vi "x410_test_host_main.vi"() -> ()   [LabVIEW 2025]
uses:
  FPGA/DataMode.ctl
  Host/Output scale.ctl
  <instrlib>/_niInstr/DSP/v1/Shared/Public/IQ Gain.ctl
  <vilib>/FPGAPlugInAG/USRP-X410/niLvFpga_Open_USRP-X410.vi
  <vilib>/rvi/interface/common/dynamic/niFpgaDynamicAddResources.vi
  <vilib>/Utility/error.llb/Error Cluster From Error Code.vi
  <vilib>/rvi/errors/niLvFpgaAdjustHostInterfaceError.vi
  <vilib>/FPGAPlugInAG/Dynamic/niLvFpga_Close_Dynamic.vi
  <vilib>/rvi/interface/nirviOpenFPGA/nirviOpenFPGA.xnode
  FPGA Bitfiles/x410_test_fpga_simple_nJrd0BX6ZCE.lvbitx
  <vilib>/rvi/interface/nirviMethod/nirviMethod.xnode
  <vilib>/rvi/interface/nirviReadWriteControl/nirviReadWriteControl.xnode
  <vilib>/rvi/interface/nirviCloseFPGA/nirviCloseFPGA.xnode
  <vilib>/rvi/errors/niLvFpgaMergeErrorWithErrorCode.vi
  NiFpgaLv.dll
  <vilib>/rvi/interface/Simulation/niFpgaSimulationCallBeginRW.vi
  <vilib>/FPGAPlugInAG/Dynamic/niLvFpga_ReadFifo_Dynamic.vi
  <instrlib>/_niInstr/DSP/v1/Shared/niInstr DSP v1 Shared.lvlib
panel:
  out "Trx Coerced Carrier Frequency":dbl format="%#_8p"
  in  "Trx Carrier Frequency":dbl format="%#_8p"
  in  "Simulated freq (kHz)":dbl
  in  "Host scale":T1
  in  "Mode":T2
  in  "Gain dB":dbl
  out "Waveform Graph":dbl[][](graph)
  out "Done":bool
  out "Init":bool
  in  "# samples to read":u32=16384
  in  "Read":bool
  in  "stop":bool
  out "Coerced Carrier Frequency":dbl=100000.0 format="%#_8p"
  in  "Carrier Frequency":dbl=2000000000.0 format="%#_8p"
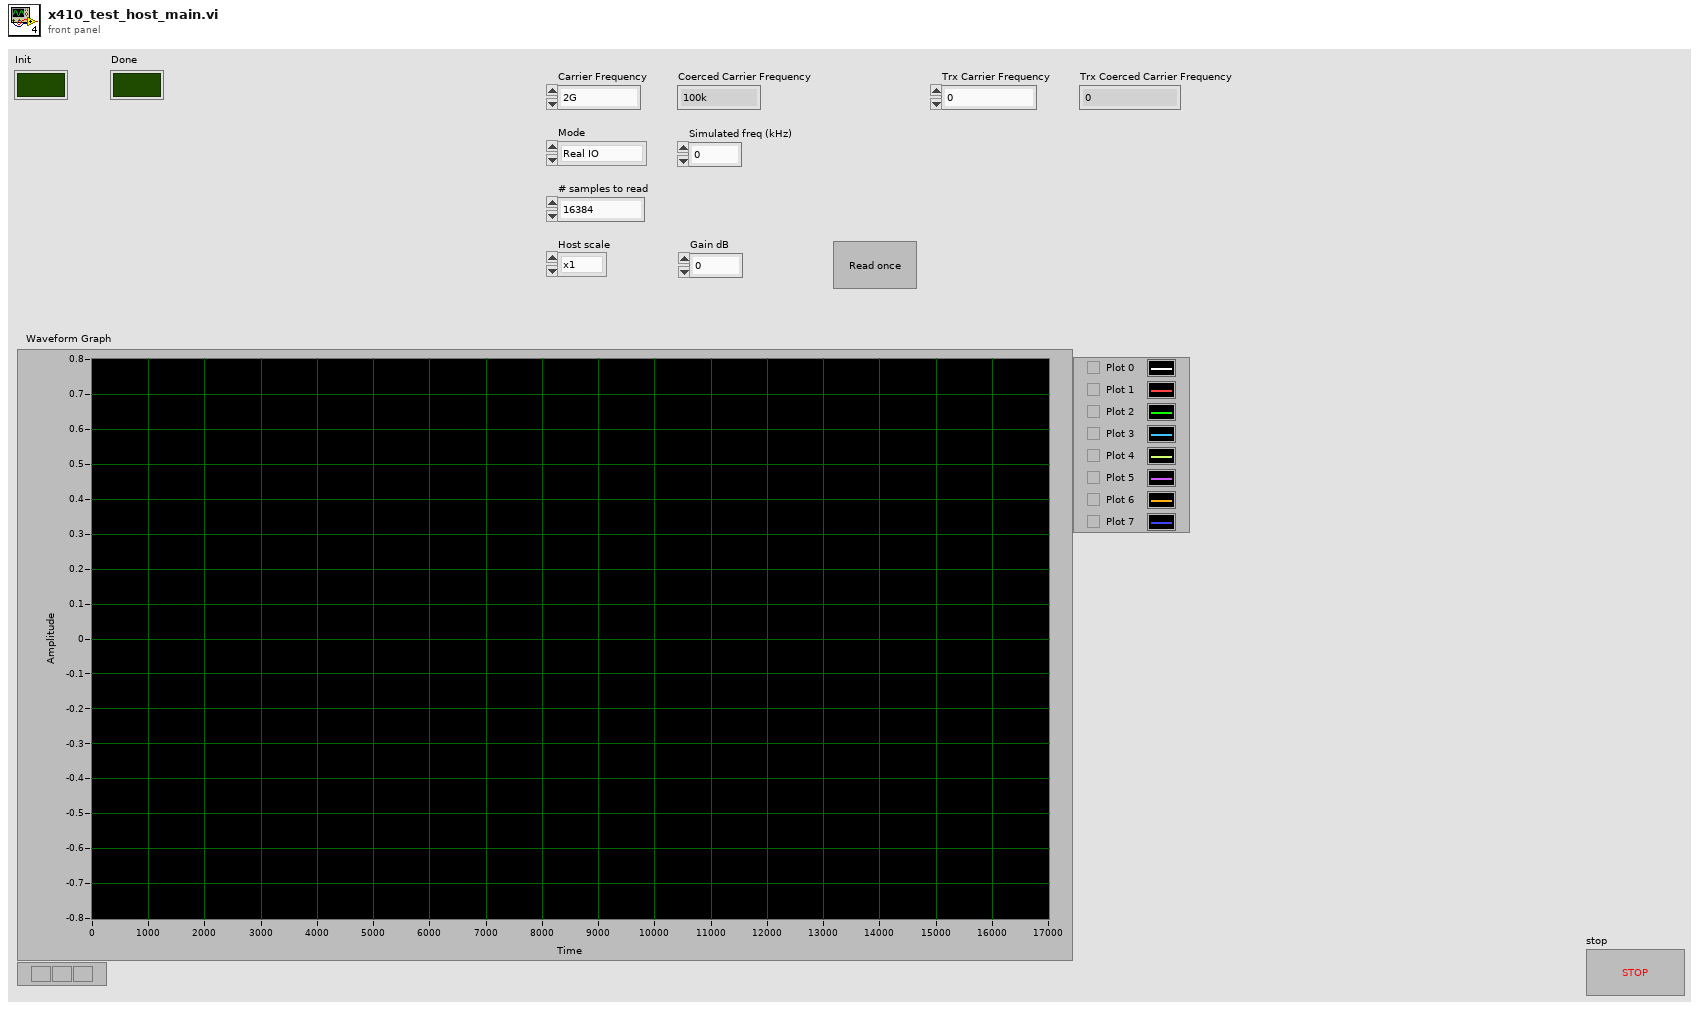
[diagram p1: front panel]
types:
  T1 = typedef "Output scale.ctl" = enum16{"x1", "x2", "x4", "x8", "x16", "x32"}
  T2 = typedef "DataMode.ctl" = enum16{"Real IO", "Simulated"}
  T3 = typedef "niInstr DSP v1 Shared.lvlib/IQ Gain.ctl" = cluster{"gain I":fxp<+/-,24,3>, "gain Q":fxp<+/-,24,3>}
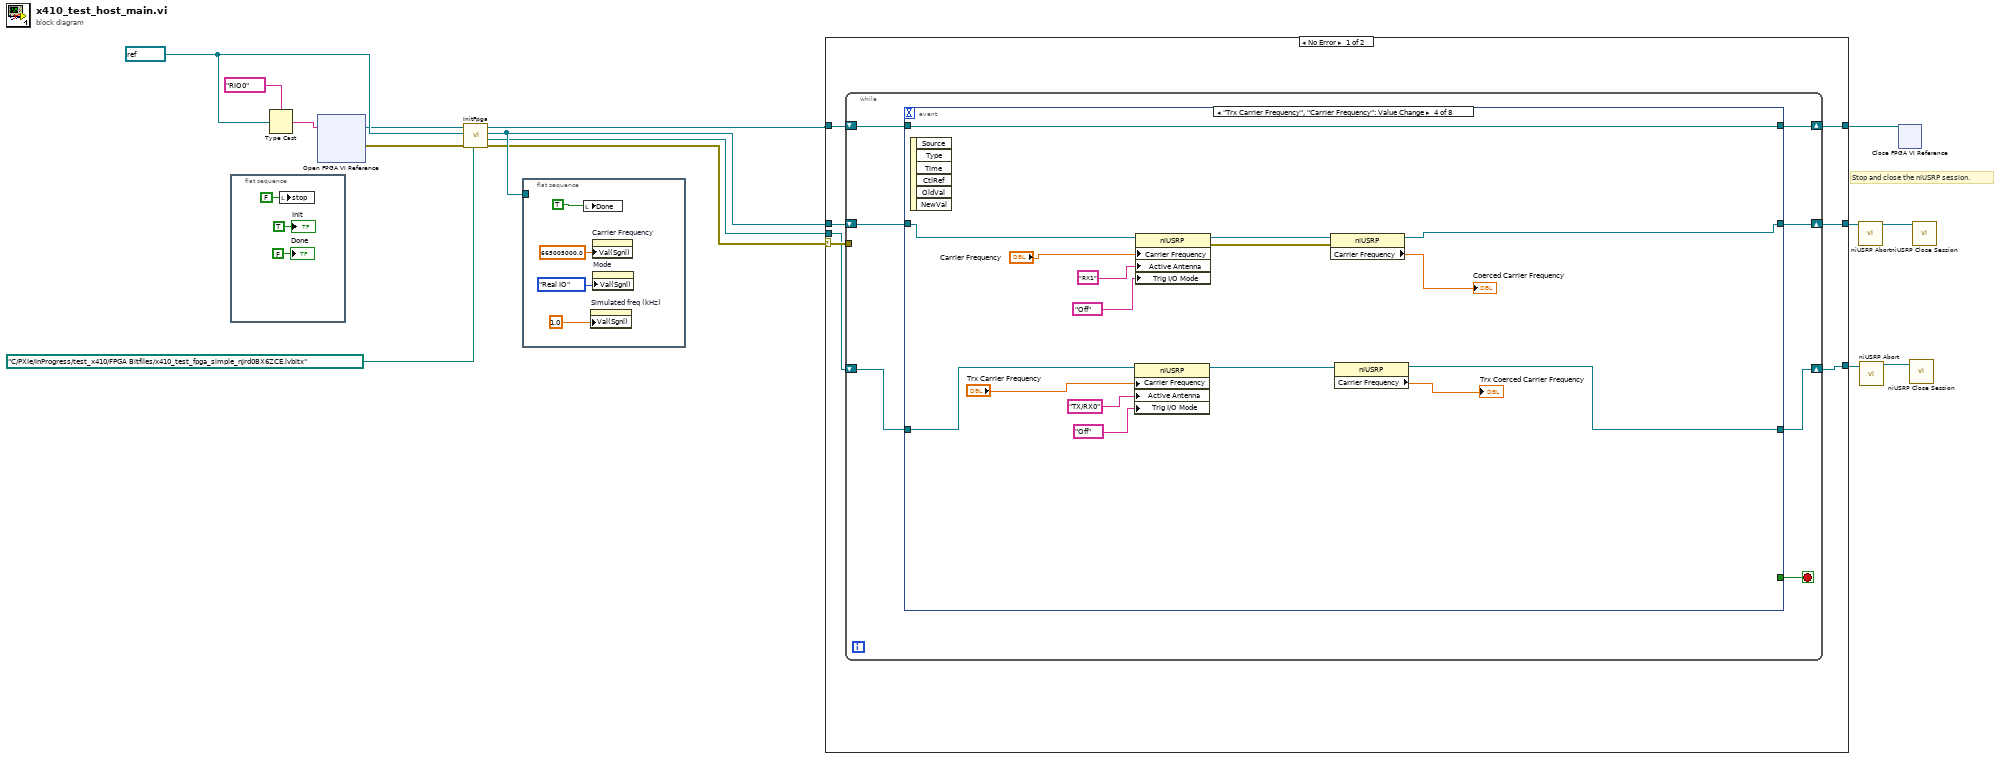
[diagram p0: block diagram]
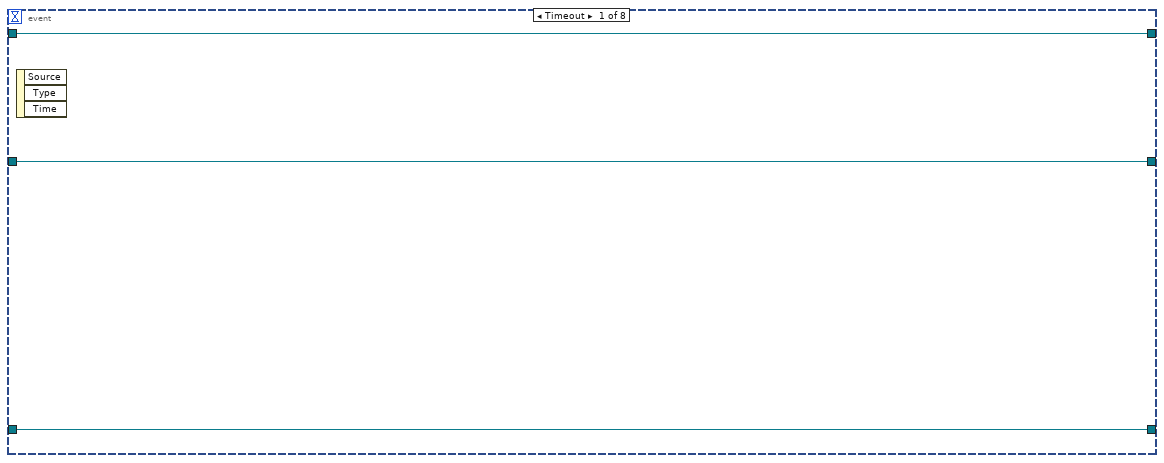
[diagram p2: hidden frame]
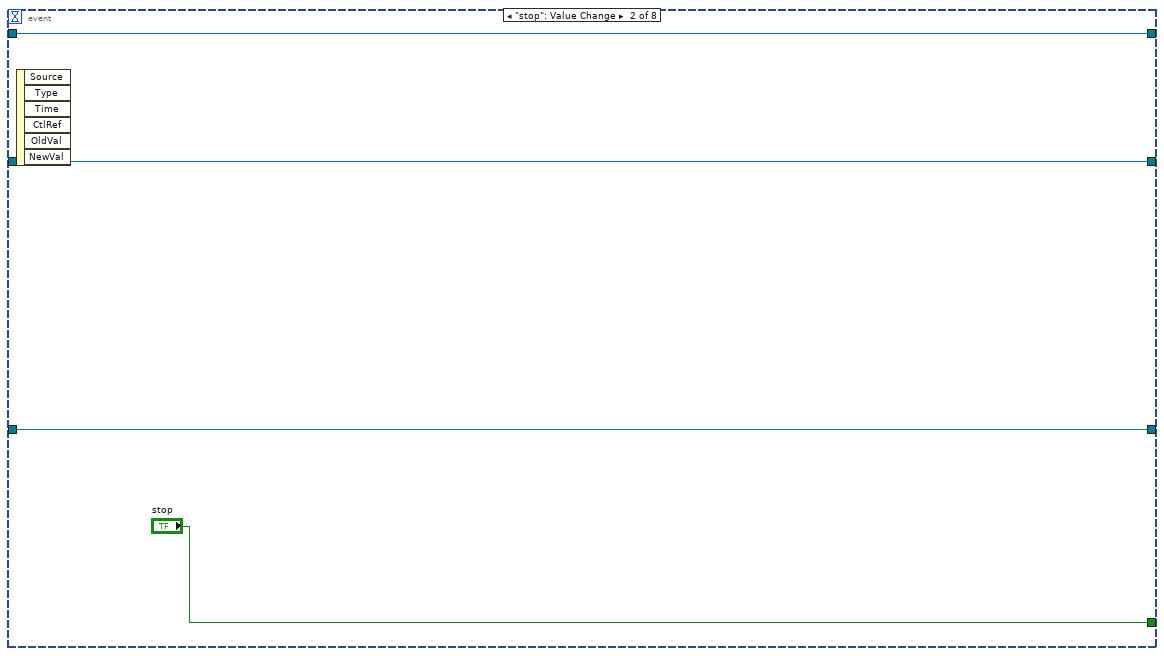
[diagram p3: hidden frame]
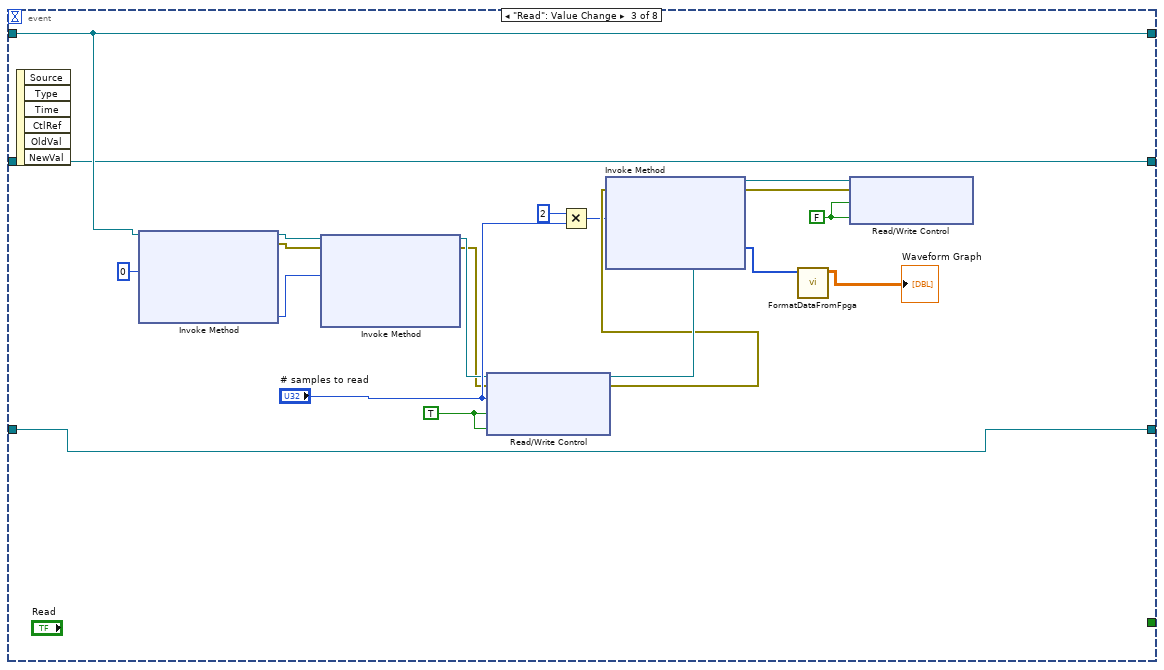
[diagram p4: hidden frame]
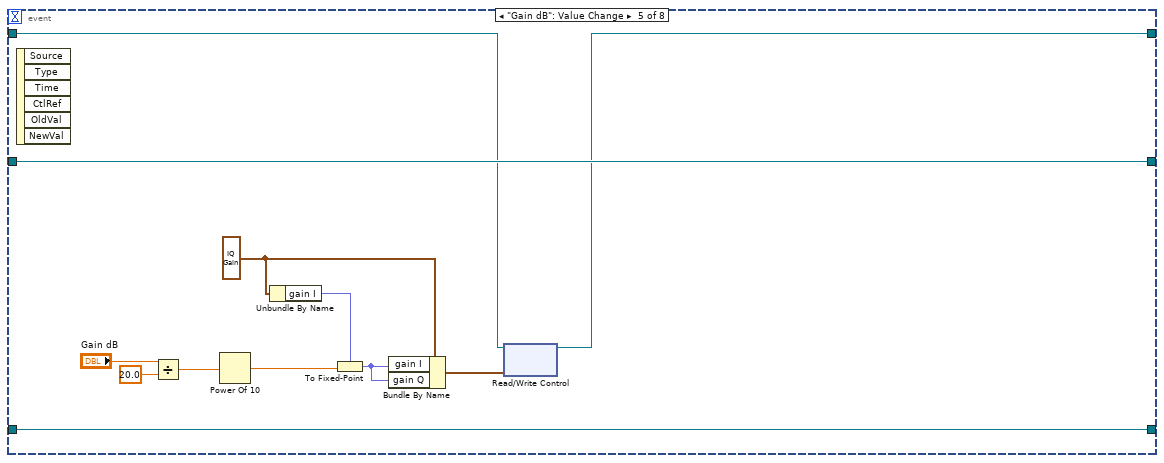
[diagram p5: hidden frame]
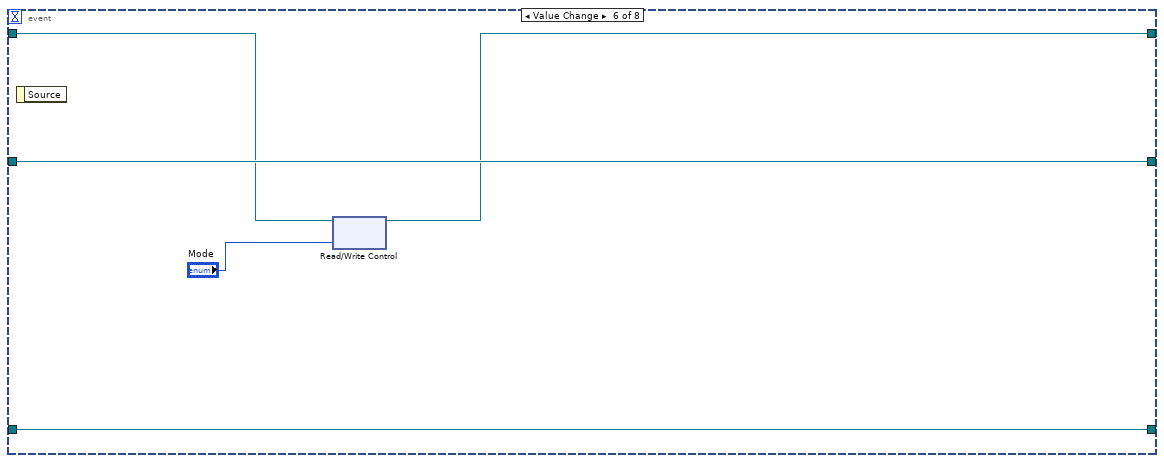
[diagram p6: hidden frame]
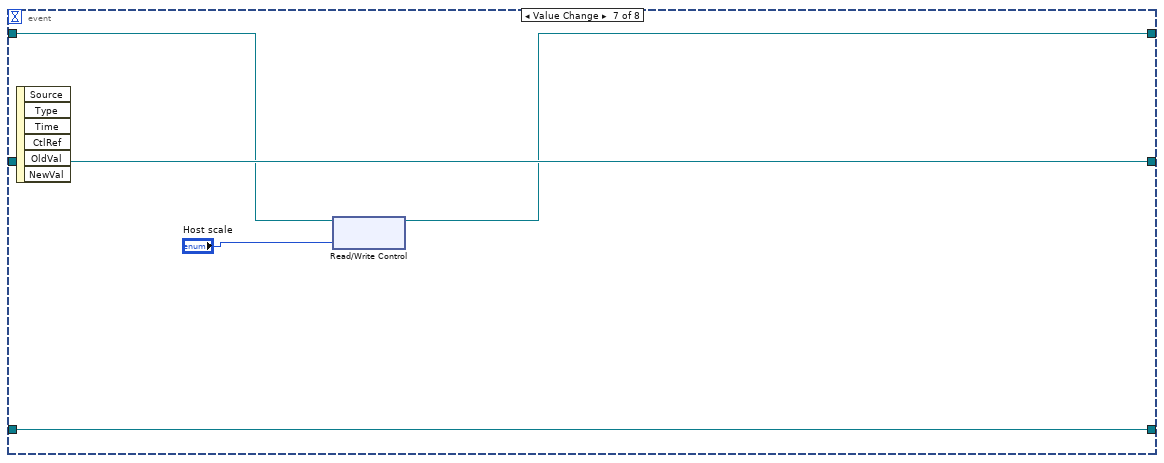
[diagram p7: hidden frame]
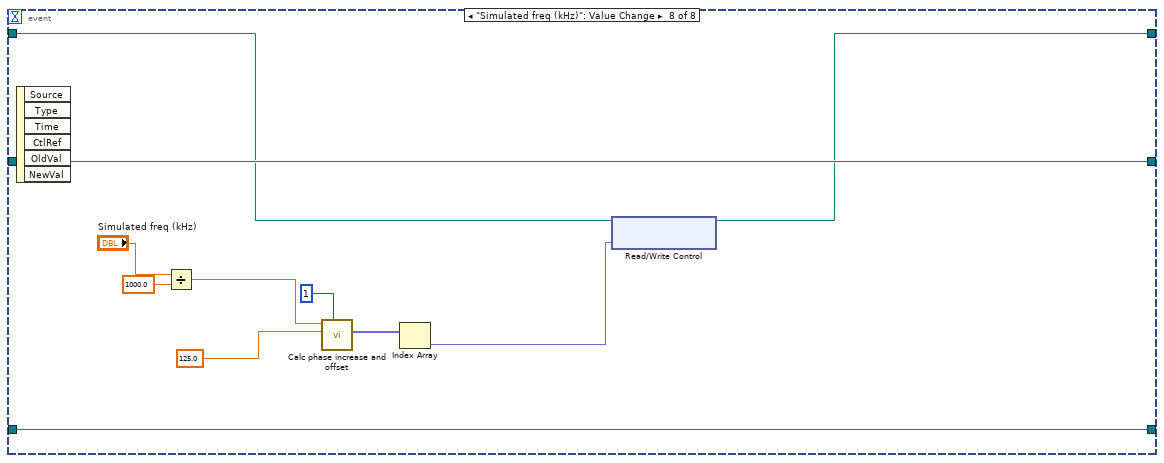
[diagram p8: hidden frame]
diagram:
  w9 = refnum<k15> "RIO0" ("Device Name")
  # "Stop and close the niUSRP session."
  n1 = flat-sequence {
    frame #0 {
      n2 = local write "stop"(FALSE ("stop")) -> ()
      "Init" <- TRUE ("Init")
      "Done" <- FALSE ("Done")
    }
  }
  n3 = Type Cast(type=tag "RIO0" ("resource name"), x=w9) -> (*(type *) &x=w12:tag)
  n4 = xnode "Open FPGA VI Reference"("resource name"=w12) -> ("FPGA VI Reference Out"=w4:refnum<k20>, "error out"=w10:errorcluster)  [unwired: 1 in]
  n5 = call "InitFpga.vi"("bitfile path"=path "C:/PXIe/InProgress/test_x410/FPGA Bitfiles/x410_test_fpga_simple_nJrd0BX6ZCE.lvbitx", "error in (no error)"=w10, "Device Name"=w9, "FPGA ref"=w4) -> ("error out"=w5:errorcluster, "session handle out 2"=w3:refnum<k15>, "session handle out"=w6:refnum<k15>, "FPGA ref out"=w7:refnum<k20>)  [unwired: 4 in]
  n6 = flat-sequence {
    tunnel: w6 -> [_]
    frame #0 {
      n7 = local write "Done"(TRUE ("Init")) -> ()
      n8 = property on="Simulated freq (kHz)" class="DigNum (strict)"("Val(Sgnl)"=1.0 ("Simulated freq (kHz)")) -> ()  [unwired: 2 in, 2 out]
      n9 = property on="Carrier Frequency" class="DigNum (strict)"("Val(Sgnl)"=665005000.0 ("Value (Signaling)")) -> ()  [unwired: 2 in, 2 out]
      n10 = property on="Mode" class="Enum (strict)"("Val(Sgnl)"=DataMode."Real IO" ("Value (Signaling)")) -> ()  [unwired: 2 in, 2 out]
    }
  }
  n11 = case shown="No Error" w5 {
    selector: w5 -> [w28 _]
    tunnel: w6 -> [w29 w115]
    tunnel: [w25 w115] -> w15
    tunnel: w7 -> [w27 w114]
    tunnel: [w26 w114] -> w13
    tunnel: w3 -> [w24 w113]
    tunnel: [w23 w113] -> w2
    frame No Error {
      n12 = while {
        tunnel: w28 -> [_]
        shift-right: [w34] -> w26
        shift-left: w27 -> [w36]
        shift-right: [w32] -> w25
        shift-left: w29 -> [w35]
        shift-right: [w30] -> w23
        shift-left: w24 -> [w31]
        stop <- w33 stop-if-true
        n13 = event shown="[3] \"Trx Carrier Frequency\", \"Carrier Frequency\": Value Change" {
          selector: _ -> [_ _ _ _ _ _ _ _]
          dyn-events: _ -> [_ _ _ _ _ _ _ _]
          timeout: _ -> [_ _ _ _ _ _ _ _]
          tunnel: w36 -> [w39 w43 w63 w79 w83 w95 w100 w111]
          tunnel: w35 -> [w38 w41 w62 w72 w91 w96 w101 w112]
          tunnel: [w39 w43 w63 w79 w82 w94 w99 w110] -> w34
          tunnel: [w38 w41 w62 w71 w91 w96 w101 w112] -> w32
          tunnel: [_ "stop" _ _ _ _ _ _] -> w33
          tunnel: w31 -> [w37 w40 w44 w70 w80 w92 w97 w102]
          tunnel: [w37 w40 w44 w64 w80 w92 w97 w102] -> w30
          event Timeout {
            n14 = event-data() -> ()  [unwired: 1 in, 3 out]
          }
          event "stop": Value Change {
            n15 = event-data() -> ()  [unwired: 1 in, 6 out]
          }
          event "Read": Value Change {
            w54 = FALSE ("Acquisition running")
            w56 = TRUE ("Acquisition running")
            n16 = event-data() -> ()  [unwired: 1 in, 6 out]
            n17 = xnode "Invoke Method"("FPGA VI Reference In"=w63, "Number of Elements"=u32 0) -> ("FPGA VI Reference Out"=w59:refnum<k20>, "error out"=w50:errorcluster, "Elements Remaining"=w58:u32)  [unwired: 2 in, 1 out]
            n18 = xnode "Invoke Method"("FPGA VI Reference In"=w59, "error in"=w50, "Number of Elements"=w58) -> ("FPGA VI Reference Out"=w57:refnum<k20>, "error out"=w49:errorcluster)  [unwired: 1 in, 2 out]
            n19 = xnode ("Read/Write Control")("FPGA VI Reference In"=w57, "error in"=w49, "Record length"="# samples to read", "Acquisition running"=w56, "Trigger Acquisition"=w56) -> ("FPGA VI Reference Out"=w55:refnum<k20>, "error out"=w48:errorcluster)
            n20 = Multiply(x=i64 2, y="# samples to read") -> (x*y=w45:i64)
            n21 = xnode "Invoke Method"("FPGA VI Reference In"=w55, "error in"=w48, "Number of Elements"=w45) -> ("FPGA VI Reference Out"=w53:refnum<k20>, "error out"=w47:errorcluster, "Data"=w52:u64[])  [unwired: 1 in, 1 out]
            n22 = call "FormatDataFromFpga.vi"("Raw data"=w52) -> ("Scaled"=→"Waveform Graph":dbl[][])  [unwired: 10 in]
            n23 = xnode "Read/Write Control"("FPGA VI Reference In"=w53, "error in"=w47, "Acquisition running"=w54, "Trigger Acquisition"=w54) -> ()  [unwired: 2 out]
          }
          event "Trx Carrier Frequency", "Carrier Frequency": Value Change {
            n24 = event-data() -> ()  [unwired: 1 in, 6 out]
            n25 = property class="niUSRP"(reference=w70, "Carrier Frequency"="Trx Carrier Frequency", "Active Antenna"="TX/RX0" ("Configuration:Active Antenna 2"), "Trig I/O Mode"="Off" ("Configuration:Trig I/O Mode")) -> (reference out=w65:refnum<k15>)  [unwired: 1 in, 1 out]
            n26 = property class="niUSRP"(reference=w72, "Carrier Frequency"="Carrier Frequency", "Active Antenna"="RX1" ("Configuration:Active Antenna"), "Trig I/O Mode"="Off" ("Configuration:Trig I/O Mode")) -> (reference out=w77:refnum<k15>, error out=w78:errorcluster)  [unwired: 1 in]
            n27 = property class="niUSRP"(reference=w77, error in=w78) -> (reference out=w71:refnum<k15>, "Carrier Frequency"=→"Coerced Carrier Frequency":dbl)  [unwired: 1 out]
            n28 = property class="niUSRP"(reference=w65) -> (reference out=w64:refnum<k15>, "Carrier Frequency"=→"Trx Coerced Carrier Frequency":dbl)  [unwired: 1 in, 1 out]
          }
          event "Gain dB": Value Change {
            w85 = T3 {"gain I"=1.0, "gain Q"=1.0} ("gain")
            n29 = event-data() -> ()  [unwired: 1 in, 6 out]
            n30 = Divide(x="Gain dB", y=20.0) -> (x/y=w88:dbl)
            n31 = Power Of 10(x=w88) -> (10^x=w87:dbl)
            n32 = Unbundle By Name(w85) -> ("gain I"=w86:fxp<+/-,24,3>)
            n33 = To Fixed-Point(fixed-point type=w86, number=w87) -> (fixed-point=w84:fxp<+/-,24,3>)
            n34 = Bundle By Name(cluster=w85, "gain I"=w84, "gain Q"=w84) -> (w81:T3)
            n35 = xnode "Read/Write Control"("FPGA VI Reference In"=w83, "gain"=w81) -> ("FPGA VI Reference Out"=w82:refnum<k20>)  [unwired: 1 in, 1 out]
          }
          event Value Change {
            n36 = event-data() -> ()  [unwired: 1 in, 1 out]
            n37 = xnode "Read/Write Control"("FPGA VI Reference In"=w95, "Mode"="Mode") -> ("FPGA VI Reference Out"=w94:refnum<k20>)  [unwired: 1 in, 1 out]
          }
          event Value Change {
            n38 = event-data() -> ()  [unwired: 1 in, 6 out]
            n39 = xnode "Read/Write Control"("FPGA VI Reference In"=w100, "Host scale"="Host scale") -> ("FPGA VI Reference Out"=w99:refnum<k20>)  [unwired: 1 in, 1 out]
          }
          event "Simulated freq (kHz)": Value Change {
            n40 = event-data() -> ()  [unwired: 1 in, 6 out]
            n41 = Divide(x="Simulated freq (kHz)", y=1000.0) -> (x/y=w104:dbl)
            n42 = call "Calc phase increase and offset.vi"("# of DDS"=1, "fclk (MHz)"=125.0, "f_generated (MHz)"=w104) -> ("Phase out"=w107:fxp<+,64,64>[])  [unwired: 6 in, 2 out]
            n43 = Index Array(array=w107) -> (element=w103:fxp<+,64,64>)  [unwired: 1 in]
            n44 = xnode "Read/Write Control"("FPGA VI Reference In"=w111, "simulated phase"=w103) -> ("FPGA VI Reference Out"=w110:refnum<k20>)  [unwired: 1 in, 1 out]
          }
        }
      }
    }
    frame Error {
    }
  }
  n45 = call <instrlib>:"niUSRP Abort.vi"("session handle"=w15) -> ("session handle out"=w14:refnum<k15>)  [unwired: 13 in, 1 out]
  n46 = call <instrlib>:"niUSRP Abort.vi"("session handle"=w2) -> ("session handle out"=w1:refnum<k15>)  [unwired: 13 in, 1 out]
  n47 = xnode "Close FPGA VI Reference"("FPGA VI Reference In"=w13) -> ()  [unwired: 1 in, 1 out]
  n48 = call <instrlib>:"niUSRP Close Session.vi"("session handle"=w1) -> ()  [unwired: 14 in, 1 out]
  n49 = call <instrlib>:"niUSRP Close Session.vi"("session handle"=w14) -> ()  [unwired: 14 in, 1 out]
